vi "Data to XY Plot RS232.vi"(7 "Input String":string) -> (8 "XY Graph":cluster{dbl[], dbl[]}(graph))   [LabVIEW 2024, in "Keithley 648X Series.lvlib"]
doc: "Sends a default command string to the instrument whenever a new VISA session is opened, or the instrument is reset. Use this VI as a subVI for the <b>Initialize</b> and <b>Reset</b> VIs. Altering this VI could cause these two VIs to operate incorrectly."
uses:
  <instrlib>/Keithley 648X Series/Keithley 648X Series.lvlib
  <vilib>/regexp/Match Regular Expression.xnode
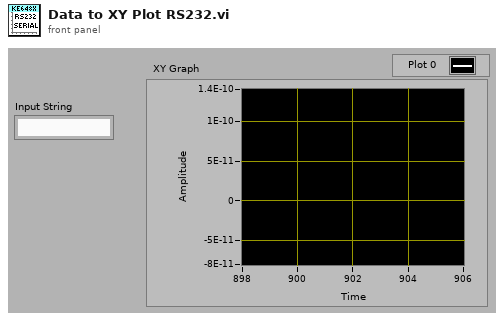
[diagram p1: front panel]
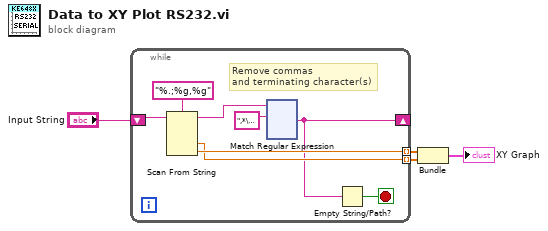
[diagram p0: block diagram]
diagram:
  n1 = while {
    shift-right: [w6] -> _
    shift-left: "Input String" -> [w11]
    tunnel: [w9] -> w4 mode=indexing
    tunnel: [w8] -> w3 mode=indexing
    stop <- w10 stop-if-true
    # "Remove commas\nand terminating character(s)"
    n2 = Scan From String(format string="%.;%g,%g", input string=w11) -> (remaining string=w5:string, output 1=w8:dbl, output 2=w9:dbl)  [unwired: 4 in, 2 out]
    n3 = xnode "Match Regular Expression"("input string"=w5, "regular expression"=",*\r*\n*\r*\n*") -> ("after match"=w6:string)  [unwired: 4 in, 4 out]
    n4 = Empty String/Path?(string/path=w6) -> (empty?=w10:bool)
  }
  n5 = Bundle(w4, w3) -> (→"XY Graph":cluster{dbl[], dbl[]})  [unwired: 1 in]
